vi "Main.vi"(0 "A":dbl, 5 "B":dbl, 7 "Stop":bool, 11 "Error in":errorcluster, 13 "Operation":enum16{"Add", "Subtract", "Multiply", "Divide"}(ring)) -> (4 "C":dbl, 15 "Error out":errorcluster)   [LabVIEW 2020, in "Simple calculator.lvlib"]
doc: "This Vi is used to implement overriding in oops in labview"
uses:
  Math Operations.lvclass
  Add.lvclass
  C:/Users/khishore.kumar/Khishore/labview_tips_2024/src/Assignment 24/Math Operations/Math Operations.lvclass
  Subtract.lvclass
  Multiply.lvclass
  Divide.lvclass
  Simple calculator.lvlib
panel:
  # "MATH OPERATIONS"
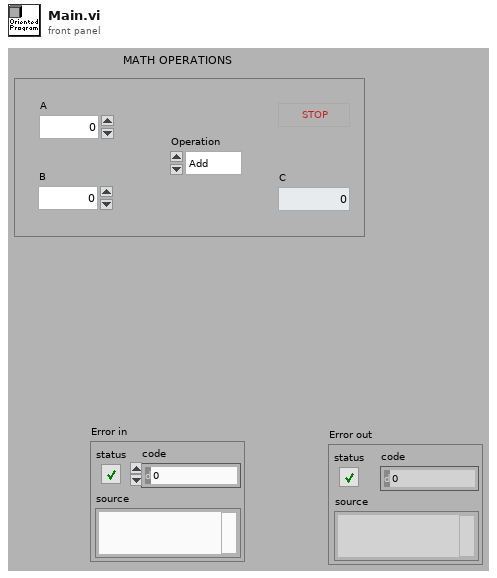
[diagram p1: front panel]
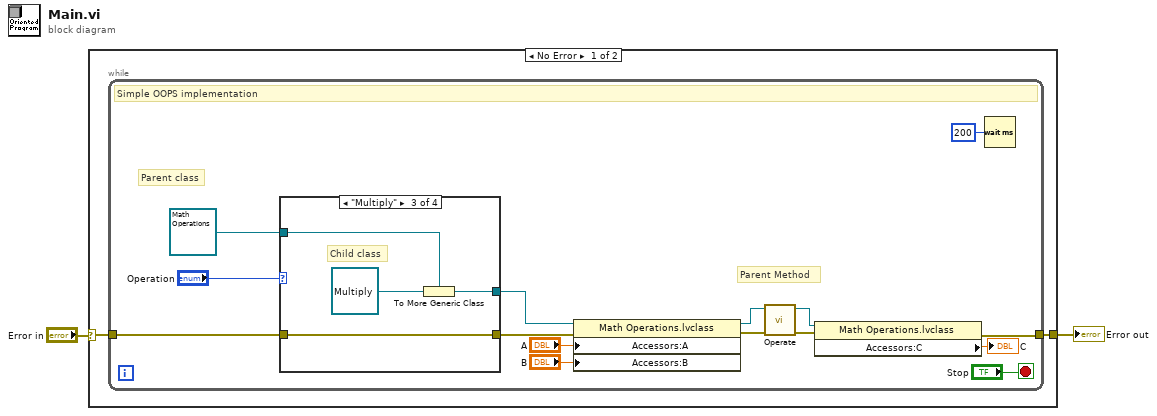
[diagram p0: block diagram]
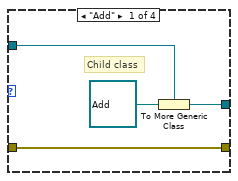
[diagram p2: hidden frame]
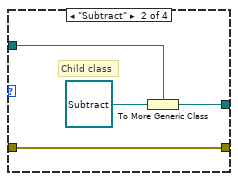
[diagram p3: hidden frame]
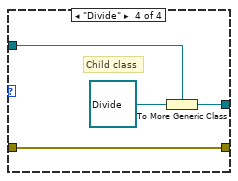
[diagram p4: hidden frame]
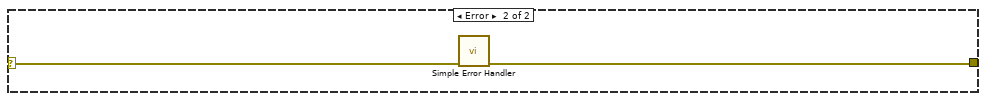
[diagram p5: hidden frame]
diagram:
  n1 = case shown="No Error" "Error in" {
    selector: "Error in" -> [w3 w37]
    tunnel: [w4 w36] -> w2
    frame No Error {
      n2 = while {
        tunnel: w3 -> [w12]
        tunnel: [w15] -> w4
        stop <- "Stop" stop-if-true
        # "Parent Method"
        # "Parent class"
        # "Simple OOPS implementation"
        n3 = case shown="\"Multiply\"" "Operation" {
          tunnel: w12 -> [w20 w27 w31 w35]
          tunnel: [w20 w27 w31 w35] -> w10
          tunnel: refnum<class "Math Operations.lvclass"> refnum ("Math Operations.lvclass") -> [w23 w24 w28 w32]
          tunnel: [w21 w25 w29 w33] -> w11
          frame "Add" {
            # "Child class"
            n4 = To More Generic Class(target class=w23, reference=refnum<class "Add.lvclass"> refnum ("Add.lvclass")) -> (generic class reference=w21:refnum<class "Math Operations.lvclass">)
          }
          frame "Subtract" {
            # "Child class"
            n5 = To More Generic Class(target class=w24, reference=refnum<class "Subtract.lvclass"> refnum ("Subtract.lvclass")) -> (generic class reference=w25:refnum<class "Math Operations.lvclass">)
          }
          frame "Multiply" {
            # "Child class"
            n6 = To More Generic Class(target class=w28, reference=refnum<class "Multiply.lvclass"> refnum ("Multiply.lvclass")) -> (generic class reference=w29:refnum<class "Math Operations.lvclass">)
          }
          frame "Divide" {
            # "Child class"
            n7 = To More Generic Class(target class=w32, reference=refnum<class "Divide.lvclass"> refnum ("Divide.lvclass")) -> (generic class reference=w33:refnum<class "Math Operations.lvclass">)
          }
        }
        n8 = property class="Math Operations.lvclass"(reference=w11, error in=w10, "Accessors:A"="A", "Accessors:B"="B") -> (reference out=w8:refnum<class "Math Operations.lvclass">, error out=w9:errorcluster)
        n9 = call-dynamic "Operate.vi"("error in (no error)"=w9, "Math Operations in"=w8) -> ("error out"=w7:errorcluster, "Math Operations out"=w6:refnum<class "Math Operations.lvclass">)  [unwired: 8 in]
        n10 = property class="Math Operations.lvclass"(reference=w6, error in=w7) -> (error out=w15:errorcluster, "Accessors:C"=→"C":dbl)  [unwired: 1 out]
        n11 = Wait (ms)(milliseconds to wait=u32 200) -> ()  [unwired: 1 out]
      }
    }
    frame Error {
      n12 = call <vilib>:"Simple Error Handler.vi"("error in (no error)"=w37) -> ("error out"=w36:errorcluster)  [unwired: 4 in, 4 out]
    }
  }
  "Error out" <- w2
